vi "Init.vi"(8 "error in (no error)":errorcluster, 10 "ID":string, 11 "Deck in":refnum<class "Deck.lvclass">) -> (0 "error out":errorcluster, 3 "Deck out":refnum<class "Deck.lvclass">)   [LabVIEW 2019, in "Deck.lvclass"]
uses:
  Deck.lvclass
  State.ctl
  Libraries/Audio Processing/Value Cluster.ctl
  Libraries/Audio Processing/Value Properties.ctl
  Libraries/Track Info/Track Info.ctl
  Deck.lvclass/Deck.ctl
  Libraries/Globals/Constants.vi
  Libraries/Audio Processing/Audio Processing.lvlib
  Libraries/Messaging/Messaging.lvlib
  Libraries/Globals/Globals.lvlib
  Libraries/Track Info/Track Info.lvlib
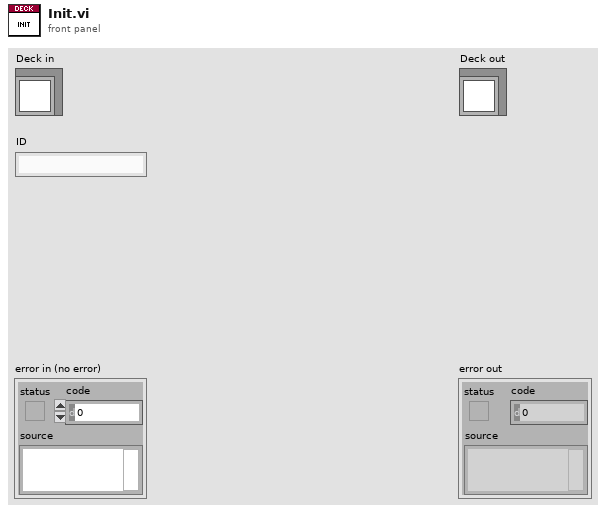
[diagram p1: front panel]
types:
  T1 = typedef "Track Info.lvlib/Track Info.ctl" = cluster{"Path":path, "Length (Samples)":i32, "Channels":i32, "Sample Rate (Hz)":i32, "BPM":dbl, "Cue Points (Samples)":i32[]}
  T2 = typedef "Audio Processing.lvlib/Value Cluster.ctl" = cluster{"Value":dbl, "Limits":T3}
  T3 = typedef "Audio Processing.lvlib/Value Properties.ctl" = cluster{"Lower":dbl, "Upper":dbl}
  T4 = typedef "Deck.lvclass/State.ctl" = enum16{"No Track", "Loading", "Active", "Scratching", "Brake", "Backspin"}
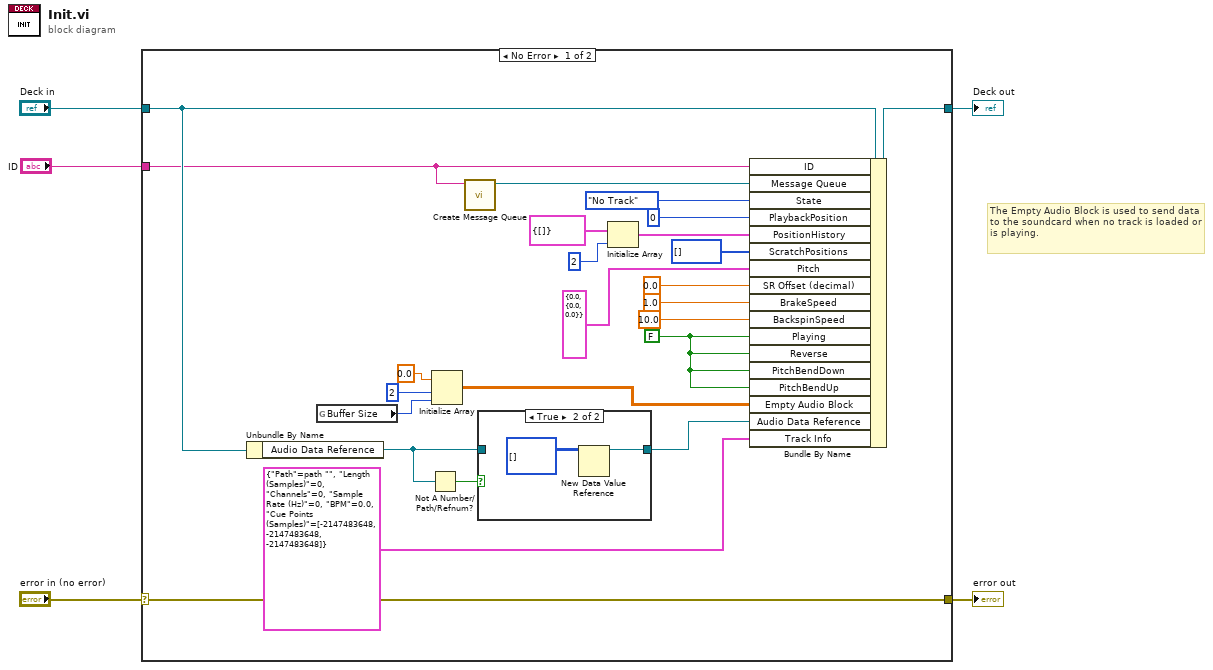
[diagram p0: block diagram]
diagram:
  # "The Empty Audio Block is used to send data to the soundcard when no track is loaded or is playing."
  n1 = case shown="No Error" "error in (no error)" {
    selector: "error in (no error)" -> [w29 w34]
    tunnel: [w29 w34] -> w4
    tunnel: [w28 w33] -> w2
    tunnel: "Deck in" -> [w23 w33]
    tunnel: "ID" -> [w10 _]
    frame No Error {
      w14 = FALSE ("PitchBendDown")
      n2 = Unbundle By Name(w23) -> ("Audio Data Reference"=w20:refnum<data-value>)
      n3 = global read "Constants.vi" "Buffer Size"() -> (w8:i32)
      n4 = Not A Number/Path/Refnum?(number/path/refnum=w20) -> (NaN/Path/Refnum?=w22:bool)
      n5 = Initialize Array(0.0, 2 ("dimension size"), w8) -> (w24:dbl[][])
      n6 = call "Create Message Queue.vi"("Queue Name"=w10) -> ("queue out"=w9:refnum<queue>)  [unwired: 9 in, 1 out]
      n7 = case shown="True" w22 {
        tunnel: [w30 w32] -> w21
        tunnel: w20 -> [w30 _]
        frame False {
        }
        frame True {
          n8 = New Data Value Reference(data value=i16[][] [] ("Audio Data")) -> (data value reference=w32:refnum<data-value>)  [unwired: 1 in, 1 out]
        }
      }
      n9 = Initialize Array(cluster{"Positions":i32[]} {"Positions"=[]} ("Cluster"), 2 ("dimension size")) -> (w16:cluster{"Positions":i32[]}[])
      n10 = Bundle By Name(cluster=w23, "ID"=w10, "Message Queue"=w9, "State"=State."No Track", "PlaybackPosition"=0 ("Playback Position (Samples)"), "PositionHistory"=w16, "ScratchPositions"=i32[] [], "Pitch"=T2 {"Value"=0.0, "Limits"={"Lower"=0.0, "Upper"=0.0}}, "SR Offset (decimal)"=0.0 ("Pitch Offset"), "BrakeSpeed"=1.0, "BackspinSpeed"=10.0, "Playing"=w14, "Reverse"=w14, "PitchBendDown"=w14, "PitchBendUp"=w14, "Empty Audio Block"=w24, "Audio Data Reference"=w21, "Track Info"=T1 {"Path"=path "", "Length (Samples)"=0, "Channels"=0, "Sample Rate (Hz)"=0, "BPM"=0.0, "Cue Points (Samples)"=[-2147483648, -2147483648, -2147483648]}) -> (w28:refnum<class "Deck.lvclass">)
    }
    frame Error {
    }
  }
  "error out" <- w4
  "Deck out" <- w2
